vi "PH_AWG-510.PC Read Settings.vi"(0 "VI in":refnum<vi>, 2 "File":string, 5 "error in (no error)":errorcluster) -> (14 "VI out":refnum<vi>, 19 "error out":errorcluster)   [LabVIEW 2014, in "PH_AWG-510.lvlib"]
doc: "This VI reads settings from harddisk to configure the hardware."
uses:
  PH_AWG-510.lvlib
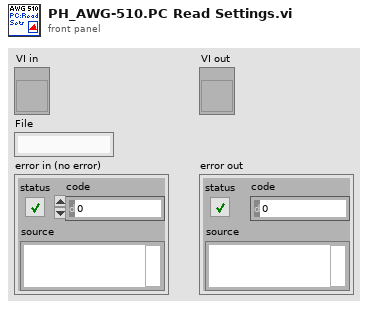
[diagram p1: front panel]
types:
  T1 = typedef "PH_AWG-510.lvlib/PH_AWG-510.i attribute.ctl" = cluster{"GUI Refs":cluster{"Delete":refnum<vi>, "Trigger Settings":refnum<vi>, "Start Device":refnum<vi>, "Instrument Information":refnum<vi>, "Lock Frontpanel":refnum<vi>, "Waveform Pattern File":refnum<vi>, "Initialize":refnum<vi>, "Output Settings":refnum<vi>}, "Instrument Information":T2, "Initialized?":bool, "Current Settings":cluster{"Trigger":T3, "Output Settings":T4}, "Wanted Settings":cluster{"Trigger":T3, "Output Settings":T4}, "Device frontpanel locked?":bool, "Default File Path":path}
  T2 = typedef "PH_AWG-510.lvlib/PH_AWG-510.Instrument Information Dataset.ctl" = cluster{"VISA resource name":refnum<visa-resource-name>, "Instrument Firmware Revision":string, "Manufacturer":string, "Model":string, "Serial Number":string, "Error Message":string, "Device Status":enum16{"stopped", "wating for trigger", "running", "Failure"}}
  T3 = typedef "PH_AWG-510.lvlib/PH_AWG-510.Trigger Settings.ctl" = cluster{"Mode":enum16{"Continuous", "Triggered", "Gated", "Enhanced"}, "Level (V)":dbl, "External Source":bool}
  T4 = typedef "PH_AWG-510.lvlib/PH_AWG-510.Output Settings.ctl" = cluster{"Activate Channel":bool, "VPP (V)":dbl, "Clock (Hz)":dbl, "File Name (Device)":string, "#1":u16, "#2":u16, "#3":u16, "#4":u16, "#5":u16, "#6":u16, "#7":u16, "#8":u16, "#9":u16, "#10":u16, "#11":u16, "#12":u16, "#13":u16, "#14":u16, "#15":u16, "#16":u16, "#17":u16, "#18":u16, "#19":u16, "#20":u16, "Offset (V)":dbl}
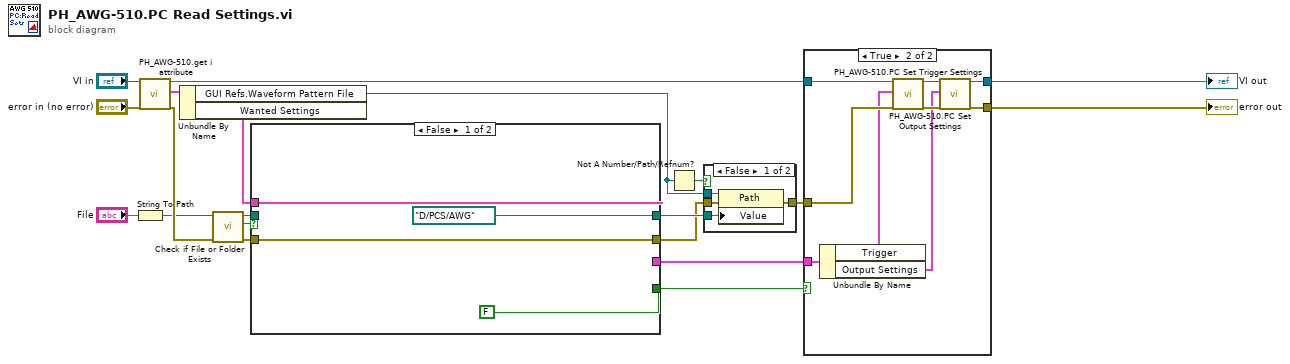
[diagram p0: block diagram]
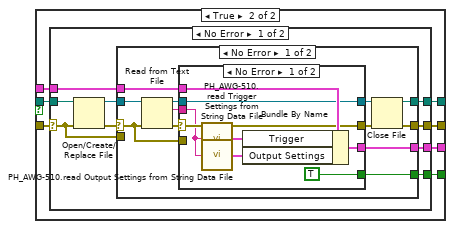
[diagram p3: hidden frame]
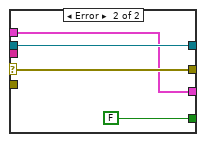
[diagram p4: hidden frame]
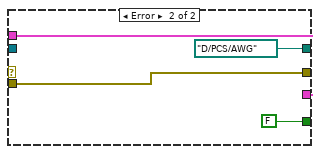
[diagram p5: hidden frame]
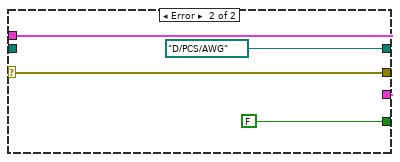
[diagram p6: hidden frame]
diagram:
  n1 = String To Path(string="File") -> (path=w1:path)
  n2 = call "PH_AWG-510.get i attribute.vi"("i ref in"="VI in", "error in (no error)"="error in (no error)") -> ("i ref out"=w14:refnum<vi>, "i attribute"=w15:T1, "error out"=w2:errorcluster)  [unwired: 15 in]
  n3 = Unbundle By Name(w15) -> ("GUI Refs.Waveform Pattern File"=w12:refnum<vi>, "Wanted Settings"=w11:cluster{"Trigger":T3, "Output Settings":T4})
  n4 = call <vilib>:"Check if File or Folder Exists.vi"("error in (no error)"=w2, "path"=w1) -> ("error out"=w9:errorcluster, "file or folder exists?"=w8:bool, "dup path"=w10:path)  [unwired: 7 in]
  n5 = case shown="False" w8 {
    tunnel: [w24 w31] -> w6
    tunnel: w9 -> [w24 w30]
    tunnel: w11 -> [w23 w29]
    tunnel: [w23 w28] -> w3
    tunnel: w10 -> [_ w27]
    tunnel: [path "D:/PCS/AWG" ("base path") w26] -> w7
    tunnel: [FALSE w25] -> w4
    frame False {
    }
    frame True {
      n6 = case shown="No Error" w30 {
        selector: w30 -> [w35 w72]
        tunnel: w27 -> [w39 _]
        tunnel: [w38 w72] -> w31
        tunnel: [w37 w71] -> w28
        tunnel: w29 -> [w34 w71]
        tunnel: [w33 path "D:/PCS/AWG" ("path")] -> w26
        tunnel: [w32 FALSE] -> w25
        frame No Error {
          n7 = Open/Create/Replace File(file path (use dialog)=w39, error in=w35) -> (refnum out=w40:refnum<file>, error out=w36:errorcluster)  [unwired: 4 in, 1 out]
          n8 = case shown="No Error" w36 {
            selector: w36 -> [w44 _]
            tunnel: w40 -> [w45 _]
            tunnel: [w49 w68] -> w38
            tunnel: [w52 w67] -> w37
            tunnel: w34 -> [w46 w67]
            tunnel: w35 -> [_ w68]
            tunnel: [w51 path "D:/PCS/AWG" ("path")] -> w33
            tunnel: [w50 FALSE] -> w32
            frame No Error {
              n9 = Read from Text File(file (use dialog)=w45, error in=w44) -> (refnum out=w41:refnum<file>, text=w43:string, error out=w42:errorcluster)  [unwired: 2 in, 1 out]
              n10 = case shown="No Error" w42 {
                selector: w42 -> [w56 _]
                tunnel: [TRUE FALSE] -> w50
                tunnel: w46 -> [w59 w61]
                tunnel: [w58 w61] -> w52
                tunnel: w43 -> [w54 _]
                tunnel: [w56 w63] -> w47
                tunnel: [w55 w62] -> w48
                tunnel: w41 -> [w55 w62]
                tunnel: w44 -> [_ w63]
                frame No Error {
                  n11 = call "PH_AWG-510.read Trigger Settings from String Data File.vi"("Data File String"=w54) -> ("Trigger Settings"=w53:T3)
                  n12 = call "PH_AWG-510.read Output Settings from String Data File.vi"("Data File String"=w54) -> ("Output Settings"=w57:T4)
                  n13 = Bundle By Name(cluster=w59, "Trigger"=w53, "Output Settings"=w57) -> (w58:cluster{"Trigger":T3, "Output Settings":T4})
                }
                frame Error {
                }
              }
              n14 = Close File(refnum=w48, error in=w47) -> (path=w51:path, error out=w49:errorcluster)
            }
            frame Error {
            }
          }
        }
        frame Error {
        }
      }
    }
  }
  n15 = Not A Number/Path/Refnum?(number/path/refnum=w12) -> (NaN/Path/Refnum?=w13:bool)
  n16 = case shown="False" w13 {
    tunnel: w6 -> [w76 w77]
    tunnel: [w75 w77] -> w5
    tunnel: w12 -> [w74 _]
    tunnel: w7 -> [w73 _]
    frame False {
      n17 = property class="Path"(reference=w74, error in=w76, "Value"=w73) -> (error out=w75:errorcluster)  [unwired: 1 out]
    }
    frame True {
    }
  }
  n18 = case shown="True" w4 {
    tunnel: w14 -> [w79 w84]
    tunnel: [w79 w88] -> w18
    tunnel: [w78 w86] -> w17
    tunnel: w5 -> [w78 w87]
    tunnel: w3 -> [_ w82]
    frame False {
    }
    frame True {
      n19 = Unbundle By Name(w82) -> ("Trigger"=w81:T3, "Output Settings"=w80:T4)
      n20 = call "PH_AWG-510.PC Set Trigger Settings.vi"("VI in"=w84, "Wanted Trigger Settings"=w81, "error in (no error)"=w87) -> ("VI out"=w83:refnum<vi>, "error out"=w85:errorcluster)  [unwired: 15 in]
      n21 = call "PH_AWG-510.PC Set Output Settings.vi"("VI in"=w83, "Wanted Output Settings"=w80, "error in (no error)"=w85) -> ("VI out"=w88:refnum<vi>, "error out"=w86:errorcluster)  [unwired: 15 in]
    }
  }
  "error out" <- w17
  "VI out" <- w18
